vi "WaitBoot.vi"(8 "error in (no error)":errorcluster, 10 "Parameters":string, 11 "reference in":refnum<class "Test_Flux_Capacitor.lvclass">) -> (0 "error out":errorcluster, 2 "Result":bool, 3 "reference out":refnum<class "Test_Flux_Capacitor.lvclass">)   [LabVIEW 2022 SP3, in "Test_Flux_Capacitor.lvlib" / "Test_Flux_Capacitor.lvclass"]
uses:
  Test_Flux_Capacitor.lvclass
  Components/Flux_Capacitor.lvlibp/Flux_Capacitor.lvclass
  <vilib>/JDP Science/JSONtext/JSONtext.lvlib
panel:
  in  "Parameter_Type":cluster{"Timeout (sec)":u32}
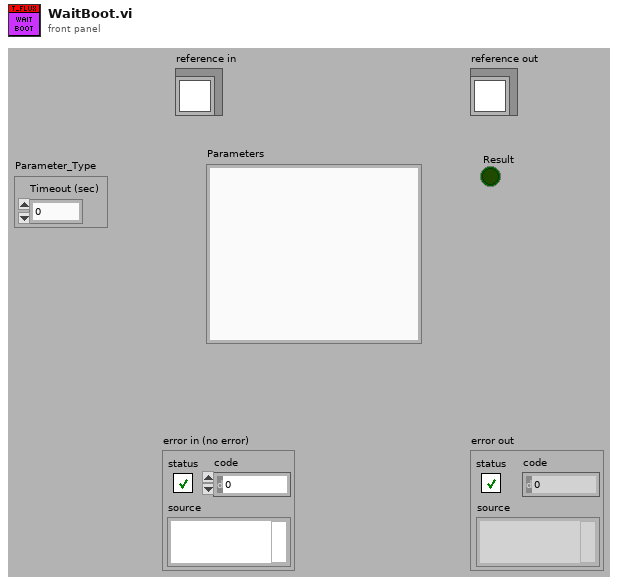
[diagram p1: front panel]
types:
  T1 = typedef "Test_Flux_Capacitor.lvlib/Test_Flux_Capacitor.lvclass/ObjectAttributes.ctl" = cluster{"Config":T2, "DMM":refnum<class "DMM_Keysight_34980A.lvclass">, "LCR":refnum<class "LCR_BK891.lvclass">, "PSU":refnum<class "PSU_Base.lvclass">, "Switch_Manager":refnum<class "SwitchBase.lvclass">, "FRAM":string, "Flux_Capacitor":refnum<class "Flux_Capacitor.lvclass">, "Frequency_Counter":refnum<class "Frequency_Counter_Base.lvclass">, "JTAG":refnum<class "JTAG_Base.lvclass">}
  T2 = typedef "Test_Flux_Capacitor.lvlib/Test_Flux_Capacitor.lvclass/Config.ctl" = cluster{"default":string}
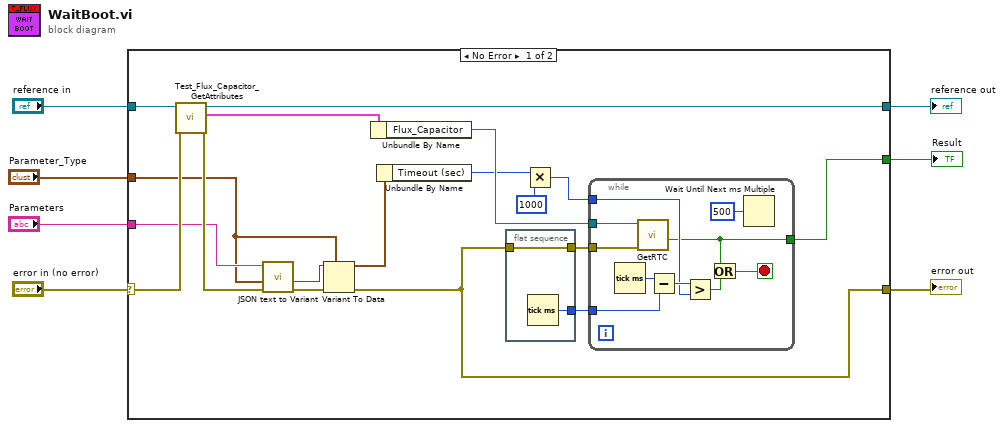
[diagram p0: block diagram]
diagram:
  n1 = case shown="No Error" "error in (no error)" {
    selector: "error in (no error)" -> [w25 w39]
    tunnel: [w17 w39] -> w6
    tunnel: [w15 w38] -> w4
    tunnel: "reference in" -> [w24 w38]
    tunnel: "Parameters" -> [w10 _]
    tunnel: "Parameter_Type" -> [w9 _]
    tunnel: [w16 _] -> w1
    frame No Error {
      n2 = call "Test_Flux_Capacitor_GetAttributes.vi"("error in (no error)"=w25, "reference in"=w24) -> ("error out"=w12:errorcluster, "Data"=w23:T1, "reference out"=w15:refnum<class "Test_Flux_Capacitor.lvclass">)  [unwired: 6 in, 1 out]
      n3 = call <vilib>:"JSON text to Variant.vi"("error in (no error)"=w12, "Data Type"=w9, "JSON"=w10) -> ("error out"=w11:errorcluster, "Variant out"=w8:variant)  [unwired: 7 in]
      n4 = Variant To Data(error in=w11, type=w9, Variant=w8) -> (data=w22:cluster{"Timeout (sec)":u32}, error out=w17:errorcluster)
      n5 = Unbundle By Name(w23) -> ("Flux_Capacitor"=w19:refnum<class "Flux_Capacitor.lvclass">)
      n6 = Unbundle By Name(w22) -> ("Timeout (sec)"=w18:u32)
      n7 = flat-sequence {
        tunnel: w17 -> [w27]
        tunnel: [w27] -> w21
        tunnel: [w26] -> w20
        frame #0 {
          n8 = Tick Count (ms)() -> (millisecond timer value=w26:u32)
        }
      }
      n9 = Multiply(x=w18, y=u32 1000) -> (x*y=w14:u32)
      n10 = while {
        tunnel: w21 -> [w36]
        tunnel: w19 -> [w37]
        tunnel: w20 -> [w34]
        tunnel: w14 -> [w29]
        tunnel: [w28] -> w16
        stop <- w31 stop-if-true
        n11 = Tick Count (ms)() -> (millisecond timer value=w35:u32)
        n12 = call-dynamic "GetRTC.vi"("error in (no error)"=w36, "reference in"=w37) -> ("OK"=w28:bool)  [unwired: 6 in, 3 out]
        n13 = Subtract(x=w35, y=w34) -> (x-y=w33:u32)
        n14 = Greater?(x=w33, y=w29) -> (0:w32:bool)
        n15 = Or(x=w28, y=w32) -> (x .or. y?=w31:bool)
        n16 = Wait Until Next ms Multiple(millisecond multiple=u32 500) -> ()  [unwired: 1 out]
      }
    }
    frame Error {
    }
  }
  "Result" <- w1
  "error out" <- w6
  "reference out" <- w4
